vi "UA Server Tests.vi"(8 "error in (no error)":errorcluster) -> (0 "error out":errorcluster)   [LabVIEW 2017, in "Unit Tests.lvlib"]
uses:
  Unit Tests.lvlib
  <vilib>/OPCUA/controls/Data Type.ctl
  <vilib>/OPCUA/controls/NodeId.ctl
  source/Browser Core/Server Classes/UA Server/Server Connection Information.ctl
  <vilib>/addons/_JKI Toolkits/Caraya/classes/Test/Test.lvclass
  <vilib>/OPCUA/NI OPC UA Server.lvlib
  <vilib>/OPCUA/NI OPC UA Utility.lvlib
  source/Browser Core/Server Classes/UA Server/UA Server.lvclass
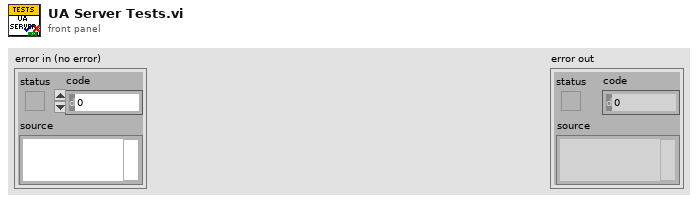
[diagram p1: front panel]
types:
  T1 = typedef "Browser Core.lvlib/UA Server.lvclass/Server Connection Information.ctl" = cluster{"Server Endpoint URL":string, "Username/Password":cluster{"Username":string, "Password":string}, "Client Certificate File":path, "Security Policy":cluster{"Message Mode":enum16{"None", "Sign", "Sign and Encrypt"}, "Security":enum16{"Basic256", "Basic128Rsa15"}}, "Trusted Server Certificates":path[]}
  T2 = typedef "Data Type.ctl" = u16
  T3 = cluster{"name":string, "data type":T2, "access level":u16, "description":string}
  T4 = typedef "NodeId.ctl" = string
  T5 = typedef "OPC UA Server Refnum.ctl" = refnum<k21>
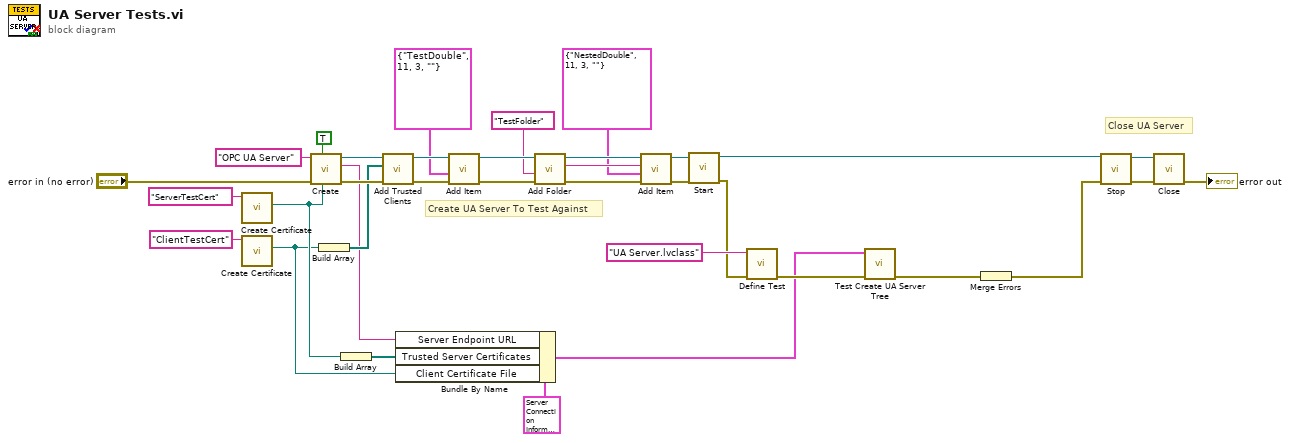
[diagram p0: block diagram]
diagram:
  # "Create UA Server To Test Against"
  # "Close UA Server"
  n1 = call <vilib>:"Create Certificate.vi"("certificate name in"="ServerTestCert") -> ("certificate path"=w9:path)  [unwired: 7 in, 3 out]
  n2 = call <vilib>:"Create Certificate.vi"("certificate name in"="ClientTestCert") -> ("certificate path"=w7:path)  [unwired: 7 in, 3 out]
  n3 = call <vilib>:"Create.vi"("server certificate file"=w9, "trust all clients (F)"=TRUE, "error in (no error)"="error in (no error)", "OPC UA server name"="OPC UA Server") -> ("error out"=w32:errorcluster, "server endpoint URL"=w6:string, "OPC UA server refnum out"=w31:T5)  [unwired: 5 in]
  n4 = Build Array(w7) -> (w28:path[])
  n5 = Build Array(w9) -> (w8:path[])
  n6 = call <vilib>:"Add Trusted Clients.vi"("error in (no error)"=w32, "trusted client certificates"=w28, "OPC UA server refnum in"=w31) -> ("error out"=w27:errorcluster, "OPC UA server refnum out"=w26:T5)  [unwired: 7 in]
  n7 = Bundle By Name(cluster=T1 {"Server Endpoint URL"="", "Username/Password"={"Username"="", "Password"=""}, "Client Certificate File"=path "", "Security Policy"={"Message Mode"=enum."None", "Security"=enum."Basic256"}, "Trusted Server Certificates"=[]} ("Server Connection Information"), "Server Endpoint URL"=w6, "Trusted Server Certificates"=w8, "Client Certificate File"=w7) -> (w2:T1)
  n8 = call <vilib>:"Add Item.vi"("error in (no error)"=w27, "item"=T3 {"name"="TestDouble", "data type"=11, "access level"=3, "description"=""}, "OPC UA server refnum in"=w26) -> ("error out"=w24:errorcluster, "OPC UA server refnum out"=w23:T5)  [unwired: 4 in, 2 out]
  n9 = call <vilib>:"Add Folder.vi"("error in (no error)"=w24, "folder name"=T4 "TestFolder" ("parent folder node ID"), "OPC UA server refnum in"=w23) -> ("error out"=w21:errorcluster, "folder node ID"=w20:T4, "OPC UA server refnum out"=w22:T5)  [unwired: 5 in]
  n10 = call <vilib>:"Add Item.vi"("error in (no error)"=w21, "item"=T3 {"name"="NestedDouble", "data type"=11, "access level"=3, "description"=""}, "parent folder node ID"=w20, "OPC UA server refnum in"=w22) -> ("error out"=w18:errorcluster, "OPC UA server refnum out"=w17:T5)  [unwired: 3 in, 2 out]
  n11 = call <vilib>:"Start.vi"("error in (no error)"=w18, "OPC UA server refnum in"=w17) -> ("error out"=w15:errorcluster, "OPC UA server refnum out"=w10:T5)  [unwired: 7 in, 1 out]
  n12 = call <vilib>:"Define Test.vi"("error in (no error)"=w15, "Label (VI Title)"="UA Server.lvclass") -> ("error out"=w4:errorcluster)  [unwired: 9 in]
  n13 = call "Test Create UA Server Tree.vi"("Error In"=w4, "Server Connection Information"=w2) -> ("Error Out"=w3:errorcluster)  [unwired: 9 in]
  n14 = Merge Errors(w3) -> (w14:errorcluster)
  n15 = call <vilib>:"Stop.vi"("error in (no error)"=w14, "OPC UA server refnum in"=w10) -> ("error out"=w13:errorcluster, "OPC UA server refnum out"=w12:T5)  [unwired: 8 in]
  n16 = call <vilib>:"Close.vi"("error in (no error)"=w13, "OPC UA server refnum in"=w12) -> ("error out"=→"error out":errorcluster)  [unwired: 9 in]
